vi "Log position.vi"(8 "error in (no error)":errorcluster, 11 "Piezo in":refnum<class "Piezo.lvclass">) -> (0 "error out":errorcluster, 3 "Piezo out":refnum<class "Piezo.lvclass">)   [LabVIEW 2012, in "Piezo.lvclass"]
uses:
  Piezo.lvclass
  Piezo.lvclass/Piezo.ctl
  <vilib>/Utility/file.llb/Write To Spreadsheet File (string).vi
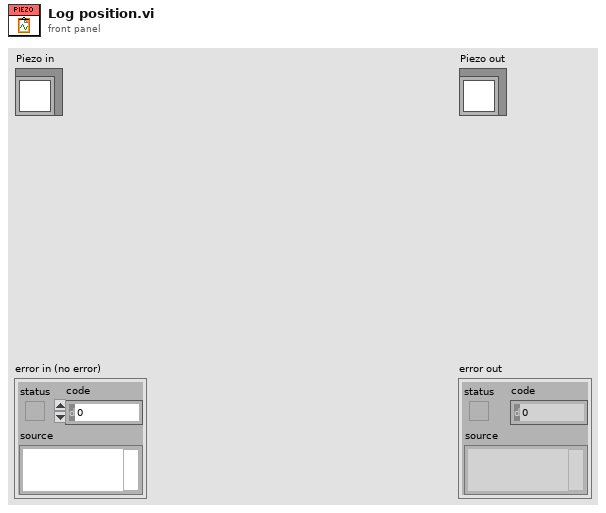
[diagram p1: front panel]
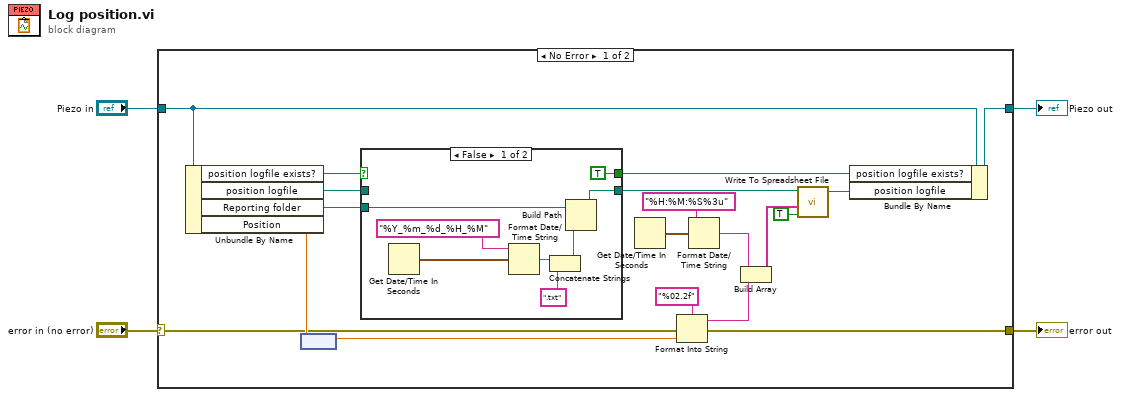
[diagram p0: block diagram]
diagram:
  n1 = case shown="No Error" "error in (no error)" {
    selector: "error in (no error)" -> [w17 w35]
    tunnel: [w16 w35] -> w3
    tunnel: [w10 w34] -> w1
    tunnel: "Piezo in" -> [w11 w34]
    frame No Error {
      n2 = Unbundle By Name(w11) -> ("position logfile exists?"=w23:bool, "position logfile"=w22:path, "Reporting folder"=w21:path, "Position"=w20:dbl[unit])
      n3 = node(w20) -> (w19:dbl)
      n4 = case shown="False" w23 {
        selector: w23 -> [_ w32]
        tunnel: w22 -> [_ w33]
        tunnel: [w29 w33] -> w15
        tunnel: w21 -> [w31 _]
        tunnel: [TRUE w32] -> w9
        frame False {
          n5 = Get Date/Time In Seconds() -> (seconds since 1Jan1904=w26:timestamp)
          n6 = Format Date/Time String(time format string (%c)="%Y_%m_%d_%H_%M", seconds (now)=w26) -> (date/time string=w27:string)  [unwired: 1 in]
          n7 = Concatenate Strings(w27, ".txt" ("string")) -> (w30:string)
          n8 = Build Path(base path=w31, name or relative path=w30) -> (appended path=w29:path)
        }
        frame True {
        }
      }
      n9 = Get Date/Time In Seconds() -> (seconds since 1Jan1904=w7:timestamp)
      n10 = Format Into String(format string="%02.2f", error in=w17, w19) -> (resulting string=w18:string, error out=w16:errorcluster)  [unwired: 1 in]
      n11 = Format Date/Time String(time format string (%c)="%H:%M:%S%3u", seconds (now)=w7) -> (date/time string=w6:string)  [unwired: 1 in]
      n12 = Build Array(w6, w18) -> (w14:string[])
      n13 = call-poly <vilib>:"Write To Spreadsheet File.vi"("append to file? (new file:F)"=TRUE, "1D data"=w14, "file path (dialog if empty)"=w15) -> ("new file path (Not A Path if cancelled)"=w8:path)  [unwired: 5 in]
      n14 = Bundle By Name(cluster=w11, "position logfile exists?"=w9, "position logfile"=w8) -> (w10:refnum<class "Piezo.lvclass">)
    }
    frame Error {
    }
  }
  "error out" <- w3
  "Piezo out" <- w1
